vi "Plat1Take.vi"(0 "StopBtnBool引用":refnum<vi>, 1 "SensorArray引用":refnum<vi>, 2 "Plat1StatueArray引用":refnum<vi>, 3 "Cmd":refnum<queue>, 4 "SolenNum_IN":refnum<queue>, 5 "SolenStatue_IN":refnum<queue>, 6 "错误输入（无错误）":errorcluster) -> (12 "错误输出":errorcluster, 17 "Cmd_OUT":refnum<queue>, 18 "SolenNum_OUT":refnum<queue>, 19 "SolenStatue_OUT":refnum<queue>)   [LabVIEW 2011]
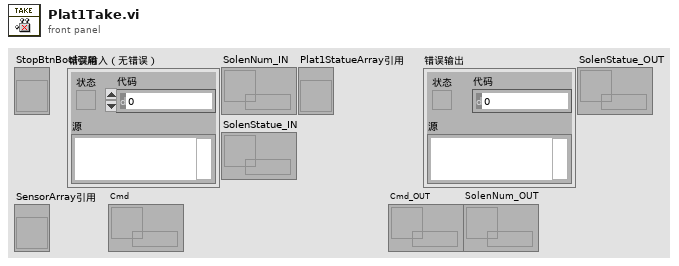
[diagram p1: front panel]
types:
  T1 = enum16{"None", "GetSensorStatue", "GetSensorAD", "GetSolenStatue", "GetPaltformStatue", "GetMotorStatue", "FeedMotorStart", "FeedMotorStop", "MotorStart", "MotorRestart", "MotorStop", "SolenAction", "SolenAdv", "RcvDataInit", "SetMotorSpeed", "Delay"}
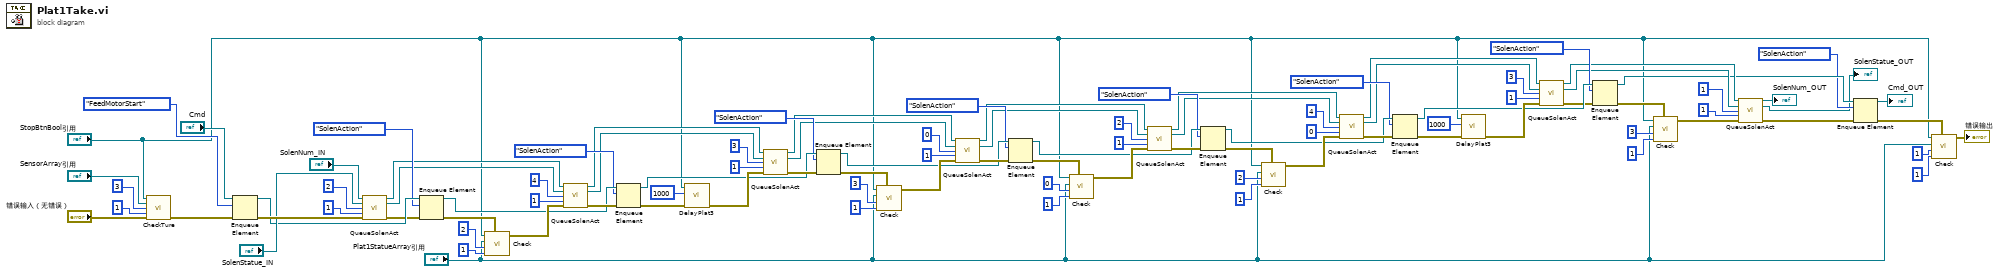
[diagram p0: block diagram]
diagram:
  n1 = call "CheckTure.vi"("Bool引用"="StopBtnBool引用", "Array引用"="SensorArray引用", "索引"=3, "长度"=1, "错误输入（无错误）"="错误输入（无错误）") -> ("错误输出"=w95:errorcluster)  [unwired: 10 in]
  n2 = Enqueue Element(queue="Cmd", element=T1."FeedMotorStart" ("元素"), error in (no error)=w95) -> (queue out=w89:refnum<queue>, error out=w92:errorcluster)  [unwired: 1 in, 1 out]
  n3 = call "QueueSolenAct.vi"("SolenNum_IN"="SolenNum_IN", "SolenStatue_IN"="SolenStatue_IN", "SolenNum_Value"=2, "SolenStatue_Value"=1, "错误输入（无错误）"=w92) -> ("SolenNum_OUT"=w80:refnum<queue>, "SolenStatue_OUT"=w79:refnum<queue>, "错误输出"=w88:errorcluster)  [unwired: 8 in]
  n4 = Enqueue Element(queue=w89, element=T1."SolenAction" ("元素"), error in (no error)=w88) -> (queue out=w75:refnum<queue>, error out=w84:errorcluster)  [unwired: 1 in, 1 out]
  n5 = call "Check.vi"("错误输入（无错误）"=w84, "长度"=1, "索引"=2, "Array引用"="Plat1StatueArray引用", "Bool引用"="StopBtnBool引用") -> ("错误输出"=w81:errorcluster)  [unwired: 6 in]
  n6 = call "QueueSolenAct.vi"("SolenNum_IN"=w80, "SolenStatue_IN"=w79, "SolenNum_Value"=4, "SolenStatue_Value"=1, "错误输入（无错误）"=w81) -> ("SolenNum_OUT"=w71:refnum<queue>, "SolenStatue_OUT"=w69:refnum<queue>, "错误输出"=w76:errorcluster)  [unwired: 8 in]
  n7 = Enqueue Element(queue=w75, element=T1."SolenAction" ("元素"), error in (no error)=w76) -> (queue out=w65:refnum<queue>, error out=w73:errorcluster)  [unwired: 1 in, 1 out]
  n8 = call "DelayPlat3.vi"("error In"=w73, "DelayTime"=u32 1000, "Bool"="StopBtnBool引用") -> ("error Out"=w70:errorcluster)  [unwired: 8 in]
  n9 = call "QueueSolenAct.vi"("SolenNum_IN"=w71, "SolenStatue_IN"=w69, "SolenNum_Value"=3, "SolenStatue_Value"=1, "错误输入（无错误）"=w70) -> ("SolenNum_OUT"=w60:refnum<queue>, "SolenStatue_OUT"=w59:refnum<queue>, "错误输出"=w66:errorcluster)  [unwired: 8 in]
  n10 = Enqueue Element(queue=w65, element=T1."SolenAction" ("元素"), error in (no error)=w66) -> (queue out=w54:refnum<queue>, error out=w63:errorcluster)  [unwired: 1 in, 1 out]
  n11 = call "Check.vi"("错误输入（无错误）"=w63, "长度"=1, "索引"=3, "Array引用"="Plat1StatueArray引用", "Bool引用"="StopBtnBool引用") -> ("错误输出"=w58:errorcluster)  [unwired: 6 in]
  n12 = call "QueueSolenAct.vi"("SolenNum_IN"=w60, "SolenStatue_IN"=w59, "SolenNum_Value"=0, "SolenStatue_Value"=1, "错误输入（无错误）"=w58) -> ("SolenNum_OUT"=w49:refnum<queue>, "SolenStatue_OUT"=w48:refnum<queue>, "错误输出"=w55:errorcluster)  [unwired: 8 in]
  n13 = Enqueue Element(queue=w54, element=T1."SolenAction" ("元素"), error in (no error)=w55) -> (queue out=w43:refnum<queue>, error out=w52:errorcluster)  [unwired: 1 in, 1 out]
  n14 = call "Check.vi"("错误输入（无错误）"=w52, "长度"=1, "索引"=0, "Array引用"="Plat1StatueArray引用", "Bool引用"="StopBtnBool引用") -> ("错误输出"=w47:errorcluster)  [unwired: 6 in]
  n15 = call "QueueSolenAct.vi"("SolenNum_IN"=w49, "SolenStatue_IN"=w48, "SolenNum_Value"=2, "SolenStatue_Value"=1, "错误输入（无错误）"=w47) -> ("SolenNum_OUT"=w37:refnum<queue>, "SolenStatue_OUT"=w36:refnum<queue>, "错误输出"=w44:errorcluster)  [unwired: 8 in]
  n16 = Enqueue Element(queue=w43, element=T1."SolenAction" ("元素"), error in (no error)=w44) -> (queue out=w32:refnum<queue>, error out=w41:errorcluster)  [unwired: 1 in, 1 out]
  n17 = call "Check.vi"("错误输入（无错误）"=w41, "长度"=1, "索引"=2, "Array引用"="Plat1StatueArray引用", "Bool引用"="StopBtnBool引用") -> ("错误输出"=w38:errorcluster)  [unwired: 6 in]
  n18 = call "QueueSolenAct.vi"("SolenNum_IN"=w37, "SolenStatue_IN"=w36, "SolenNum_Value"=4, "SolenStatue_Value"=0, "错误输入（无错误）"=w38) -> ("SolenNum_OUT"=w27:refnum<queue>, "SolenStatue_OUT"=w26:refnum<queue>, "错误输出"=w33:errorcluster)  [unwired: 8 in]
  n19 = Enqueue Element(queue=w32, element=T1."SolenAction" ("元素"), error in (no error)=w33) -> (queue out=w23:refnum<queue>, error out=w30:errorcluster)  [unwired: 1 in, 1 out]
  n20 = call "DelayPlat3.vi"("error In"=w30, "DelayTime"=u32 1000, "Bool"="StopBtnBool引用") -> ("error Out"=w28:errorcluster)  [unwired: 8 in]
  n21 = call "QueueSolenAct.vi"("SolenNum_IN"=w27, "SolenStatue_IN"=w26, "SolenNum_Value"=3, "SolenStatue_Value"=1, "错误输入（无错误）"=w28) -> ("SolenNum_OUT"=w17:refnum<queue>, "SolenStatue_OUT"=w16:refnum<queue>, "错误输出"=w22:errorcluster)  [unwired: 8 in]
  n22 = Enqueue Element(queue=w23, element=T1."SolenAction" ("元素"), error in (no error)=w22) -> (queue out=w11:refnum<queue>, error out=w20:errorcluster)  [unwired: 1 in, 1 out]
  n23 = call "Check.vi"("错误输入（无错误）"=w20, "长度"=1, "索引"=3, "Array引用"="Plat1StatueArray引用", "Bool引用"="StopBtnBool引用") -> ("错误输出"=w15:errorcluster)  [unwired: 6 in]
  n24 = call "QueueSolenAct.vi"("SolenNum_IN"=w17, "SolenStatue_IN"=w16, "SolenNum_Value"=1, "SolenStatue_Value"=1, "错误输入（无错误）"=w15) -> ("SolenNum_OUT"=→"SolenNum_OUT":refnum<queue>, "SolenStatue_OUT"=→"SolenStatue_OUT":refnum<queue>, "错误输出"=w12:errorcluster)  [unwired: 8 in]
  n25 = Enqueue Element(queue=w11, element=T1."SolenAction" ("元素"), error in (no error)=w12) -> (queue out=→"Cmd_OUT":refnum<queue>, error out=w9:errorcluster)  [unwired: 1 in, 1 out]
  n26 = call "Check.vi"("错误输入（无错误）"=w9, "长度"=1, "索引"=1, "Array引用"="Plat1StatueArray引用", "Bool引用"="StopBtnBool引用") -> ("错误输出"=→"错误输出":errorcluster)  [unwired: 6 in]
